vi "Initialise.vi"(8 "error in (no error)":errorcluster) -> (0 "error out":errorcluster, 3 "Elapsed Time out":refnum<class "Elapsed Time.lvclass">)   [LabVIEW 2015, in "Elapsed Time.lvclass"]
doc: "Resets the Elapsed time."
uses:
  Elapsed Time.lvclass
  Elapsed Time.lvclass/Elapsed Time.ctl
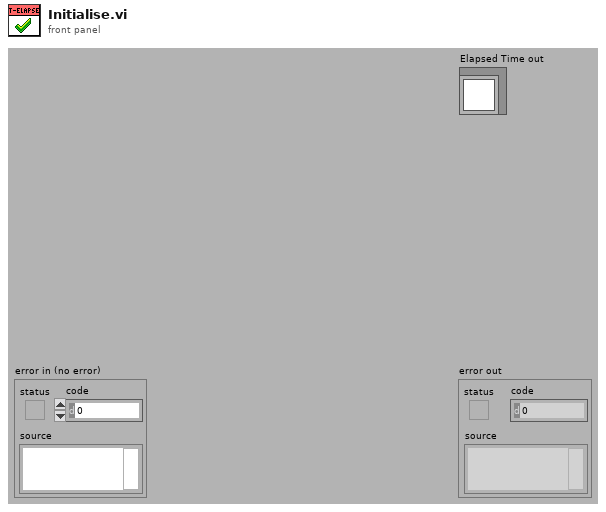
[diagram p1: front panel]
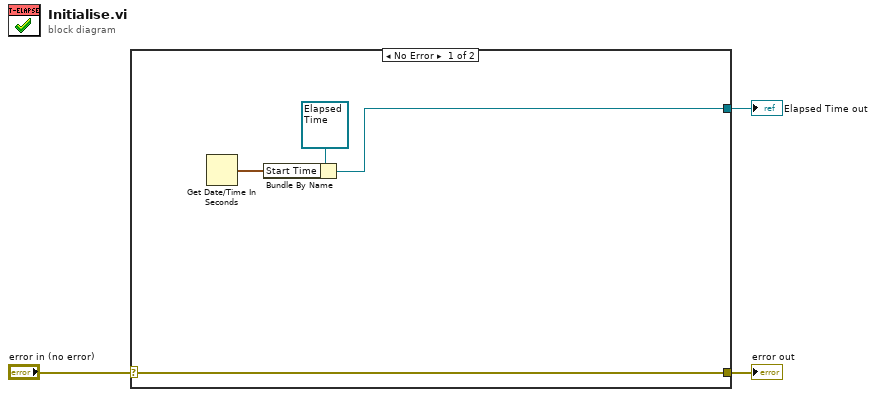
[diagram p0: block diagram]
diagram:
  n1 = case shown="No Error" "error in (no error)" {
    selector: "error in (no error)" -> [w7 w8]
    tunnel: [w7 w8] -> w2
    tunnel: [w5 _] -> w1
    frame No Error {
      n2 = Get Date/Time In Seconds() -> (seconds since 1Jan1904=w4:timestamp)
      n3 = Bundle By Name(cluster=refnum<class "Elapsed Time.lvclass"> refnum ("Elapsed Time.lvclass"), "Start Time"=w4) -> (w5:refnum<class "Elapsed Time.lvclass">)
    }
    frame Error {
    }
  }
  "error out" <- w2
  "Elapsed Time out" <- w1
